vi "Simple AAP.vi"() -> ()   [LabVIEW 2015]
panel:
  out "Waveform Graph":dynamicdata(graph)
  out "Avarage Value":dbl
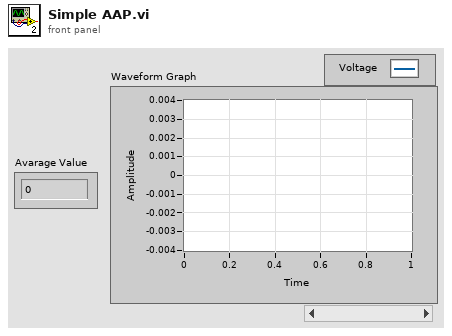
[diagram p1: front panel]
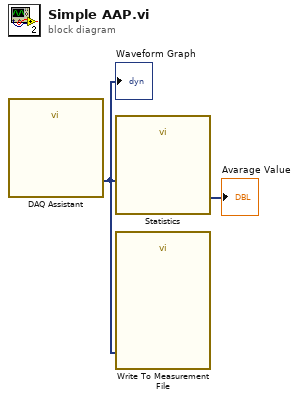
[diagram p0: block diagram]
diagram:
  n1 = call "DAQ Assistant"() -> ("data"=w2:dynamicdata)  [unwired: 17 in, 2 out]
  "Waveform Graph" <- w2
  n2 = call "Statistics"("Signals"=w2) -> ("Arithmetic Mean"=→"Avarage Value":dynamicdata)  [unwired: 25 in, 1 out]
  n3 = call "Write To Measurement File"("Signals"=w2) -> ()  [unwired: 16 in, 3 out]
